vi "load, grow blob.vi"() -> ()   [LabVIEW 2011]
uses:
  <userlib>/labvvis/New Image/New Image (Grey).vi
  <userlib>/labvvis/labvvis.lvlib
panel:
  out "Input":picture
  out "Error":string
  in  "path to JPEG file":path
  out "Output":picture
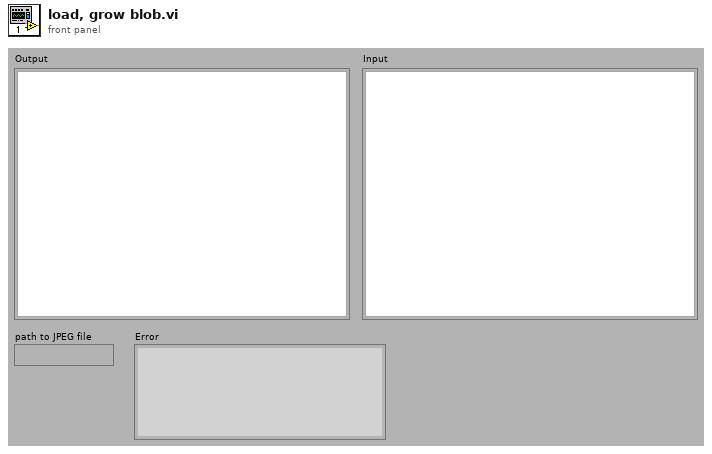
[diagram p1: front panel]
types:
  T1 = typedef "imagedata.ctl" = cluster{"image type":i32, "image depth":i32, "image":u8[], "mask":u8[], "colors":u32[], "Rectangle":cluster{"left":i16, "top":i16, "right":i16, "bottom":i16}}
  T2 = typedef "labvvis.lvlib/VVIS Image.ctl" = cluster{"Image ID":i16, "Channel ID":i16}
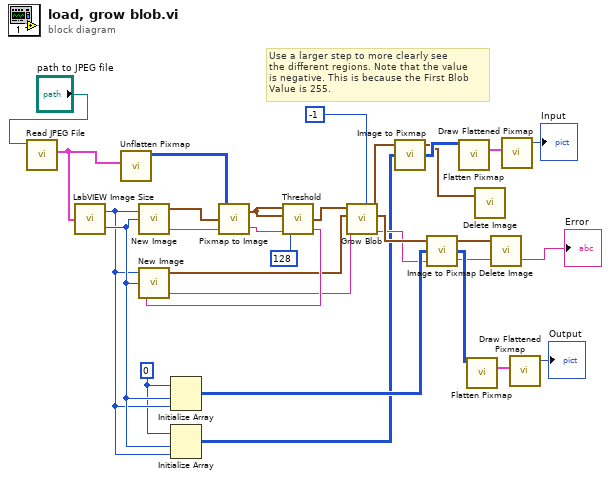
[diagram p0: block diagram]
diagram:
  w9 = 0
  # "Use a larger step to more clearly see\nthe different regions. Note that the value \nis negative. This is because the First Blob\nValue is 255."
  n1 = call <vilib>:"Read JPEG File.vi"("path to JPEG file"="path to JPEG file") -> ("image data"=w20:T1)  [unwired: 8 in, 2 out]
  n2 = call <userlib>:"LabVIEW Image Size.vi"("Cluster"=w20) -> ("Width"=w10:i16, "Height"=w11:i16)
  n3 = call <vilib>:"Unflatten Pixmap.vi"("image data"=w20) -> ("24-bit pixmap"=w27:u32[][])  [unwired: 4 in, 6 out]
  n4 = call-poly <userlib>:"New Image.vi"("Height"=w11, "Width"=w10) -> ("Error"=w21:string, "VVIS Image"=w28:T2)  [unwired: 2 in]
  n5 = Initialize Array(w9, w11, w10) -> (w25:i32[][])
  n6 = Initialize Array(w9, w11, w10) -> (w8:i32[][])
  n7 = call <userlib>:"Pixmap to Image.vi"("Error"=w21, "Output Image"=w28, "Input Pixmap"=w27) -> ("Error"=w16:string, "Output Image"=w19:T2)
  n8 = call <userlib>:"Threshold.vi"("Error"=w16, "Threshold"=i16 128, "Output Image"=w19, "Input Image"=w19) -> ("Error"=w17:string, "Output Image"=w7:T2)  [unwired: 1 out]
  n9 = call-poly <userlib>:"New Image.vi"("Error"=w17, "Height"=w11, "Width"=w10) -> ("Error"=w12:string, "VVIS Image"=w15:T2)  [unwired: 1 in]
  n10 = call <userlib>:"Grow Blob.vi"("Blob Step"=i16 -1, "Error"=w12, "Output Image"=w15, "Input Image"=w7) -> ("Error"=w13:string, "Output Image"=w14:T2, "Input Image"=w3:T2)  [unwired: 3 in]
  n11 = call <userlib>:"Image to Pixmap.vi"("Output Pixmap"=w8, "Image"=w3) -> ("Output Pixmap"=w4:u32[][], "Image"=w2:T2)  [unwired: 1 in, 1 out]
  n12 = call <userlib>:"Image to Pixmap.vi"("Error"=w13, "Output Pixmap"=w25, "Image"=w14) -> ("Error"=w23:string, "Output Pixmap"=w26:u32[][], "Image"=w24:T2)
  n13 = call <vilib>:"Flatten Pixmap.vi"("24-bit pixmap"=w4) -> ("image data"=w5:T1)  [unwired: 10 in]
  n14 = call <vilib>:"Flatten Pixmap.vi"("24-bit pixmap"=w26) -> ("image data"=w29:T1)  [unwired: 10 in]
  n15 = call <userlib>:"Delete Image.vi"("Image"=w2) -> ()  [unwired: 2 in, 1 out]
  n16 = call <userlib>:"Delete Image.vi"("Error"=w23, "Image"=w24) -> ("Error"=→"Error":string)  [unwired: 1 in]
  n17 = call <vilib>:"Draw Flattened Pixmap.vi"("image data"=w5) -> ("new picture"=→"Input":picture)  [unwired: 8 in]
  n18 = call <vilib>:"Draw Flattened Pixmap.vi"("image data"=w29) -> ("new picture"=→"Output":picture)  [unwired: 8 in]
